vi "Read Error Report.vi"(8 "error in (no error)":errorcluster, 11 "Last Ack in":refnum<class "Last Ack.lvclass">) -> (0 "error out":errorcluster, 3 "Error Report":errorcluster)   [LabVIEW 2016, in "Stream Mediator.lvlib" / "Last Ack.lvclass"]
doc: "--\nCopyright © 2017 Composed SystemsI All rights reserved.\n\nAuthor: Jon McBee <jon.mcbee@composed.io>\n\nThis library is provided \"AS IS\" ,WITHOUT WARRANTIES OR\nCONDITIONS OF ANY KIND, either express or implied.\n\nComposed Systems -- composed.io\n\nStream 0.0.1.1\nJon McBee - Composed Systems\nCopyright (c) 2017, Composed Systems"
uses:
  <userlib>/Composed Systems/Stream/Mediator/Classes/Message Command Last Ack/Last Ack.lvclass
  <userlib>/Composed Systems/Stream/Mediator/Classes/Message Command Last Ack/Last Ack.lvclass/Last Ack.ctl
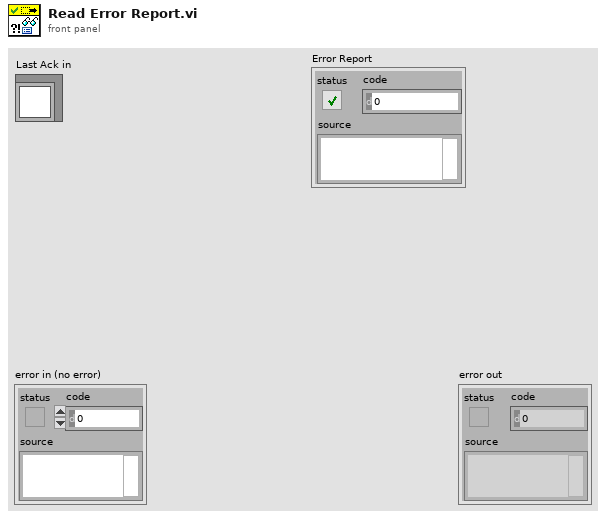
[diagram p1: front panel]
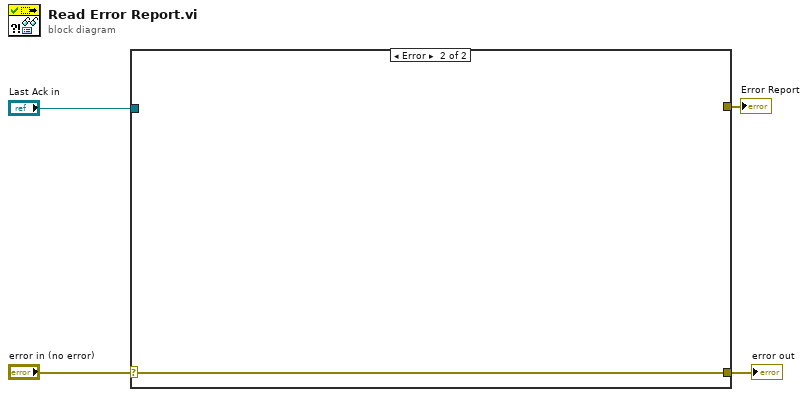
[diagram p0: block diagram]
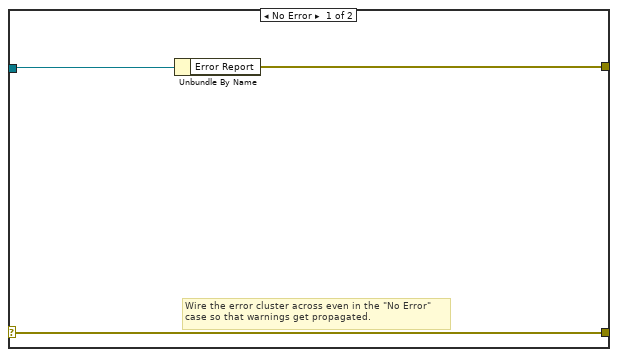
[diagram p2: hidden frame]
diagram:
  n1 = case shown="Error" "error in (no error)" {
    selector: "error in (no error)" -> [w7 w8]
    tunnel: [w7 w8] -> w3
    tunnel: "Last Ack in" -> [w6 _]
    tunnel: [w5 _] -> w1
    frame No Error {
      # "Wire the error cluster across even in the \"No Error\"\ncase so that warnings get propagated."
      n2 = Unbundle By Name(w6) -> ("Error Report"=w5:errorcluster)
    }
    frame Error {
    }
  }
  "error out" <- w3
  "Error Report" <- w1
